vi "RPC Method Query.vi"(8 "error in (no error)":errorcluster, 11 "OOP Server in":refnum<class "Query Server.lvclass">) -> (0 "error out":errorcluster, 3 "OOP Server out":refnum<class "Query Server.lvclass">)   [LabVIEW 2016, in "Query Server.lvlib" / "Query Server.lvclass"]
uses:
  Query Server.lvclass
  RPC Messages/QueryResponse/QueryResponse_Data.ctl
panel:
  out "State Data":string
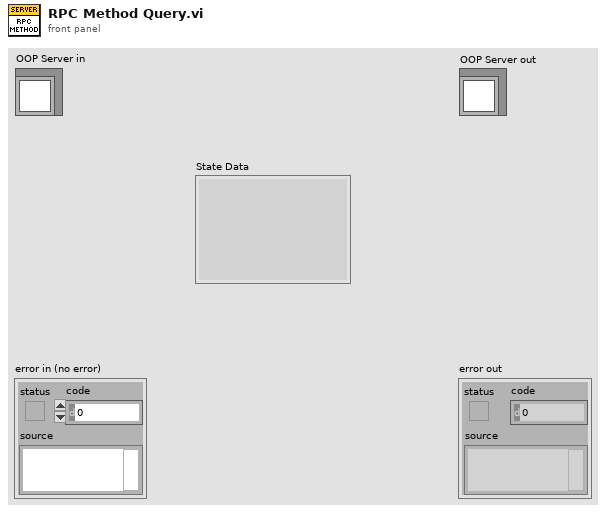
[diagram p1: front panel]
types:
  T1 = typedef "Query Server.lvlib/Query Server.lvclass/QueryResponse_Data.ctl" = cluster{"message":string, "status":i32}
  T2 = typedef "Query Server.lvlib/Query Server.lvclass/Server Internal UEs.ctl" = cluster{"Invoke Internal UE":refnum<user-event>, "Query Internal UE":refnum<user-event>, "Register Internal UE":refnum<user-event>}
  T3 = typedef "Query Server.lvlib/Query Server.lvclass/Server gRPC UEs.ctl" = cluster{"Invoke gRPC UE":refnum<user-event>, "Query gRPC UE":refnum<user-event>, "Register gRPC UE":refnum<user-event>}
  T4 = typedef "Query Server.lvlib/gprc-lvsupport.lvlib/grpcId.ctl" = u64
  T5 = typedef "Query Server.lvlib/Query Server.lvclass/QueryRequest_Data.ctl" = cluster{"query":string}
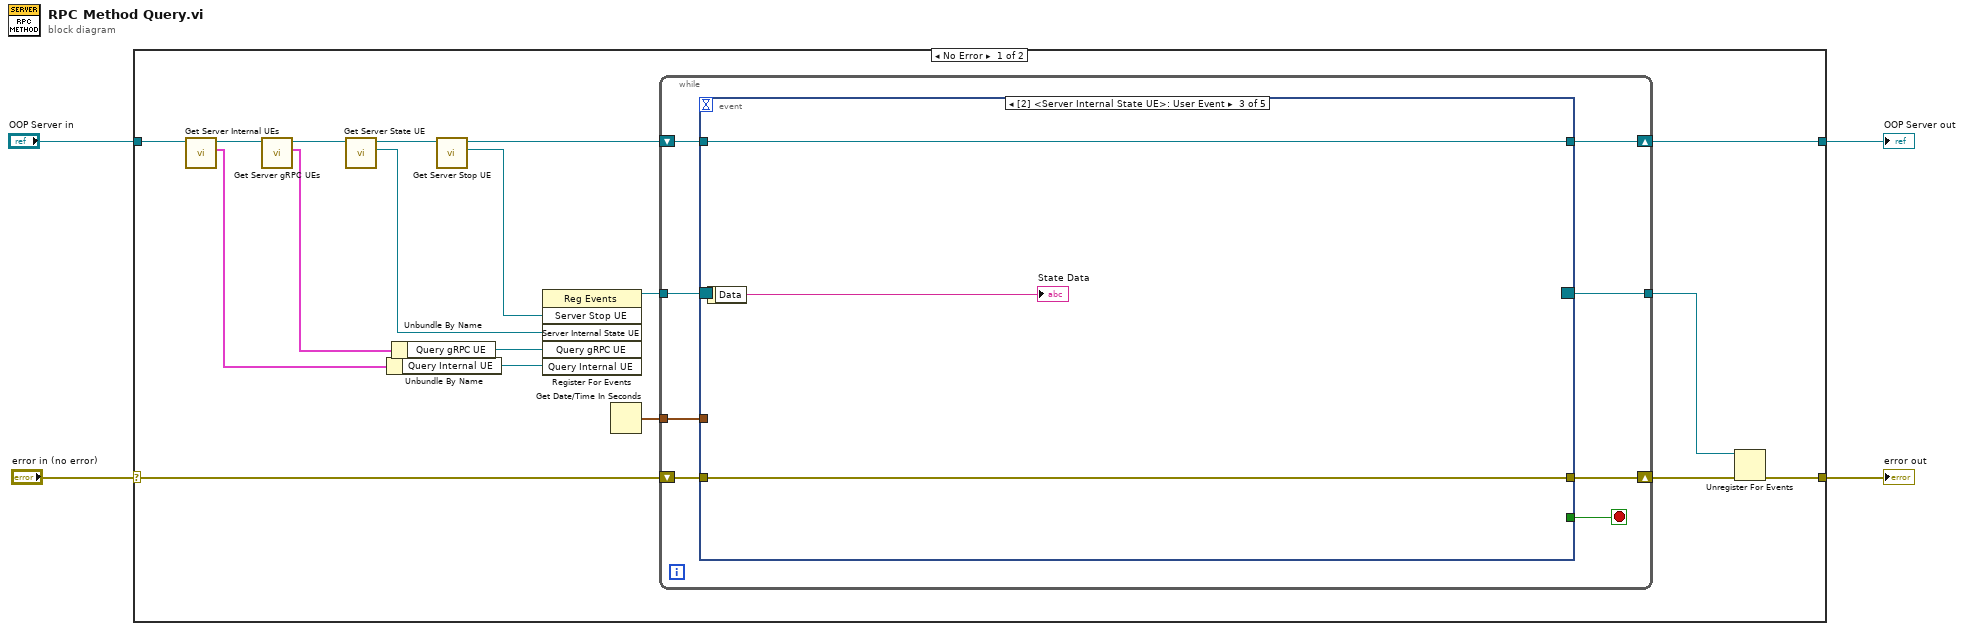
[diagram p0: block diagram]
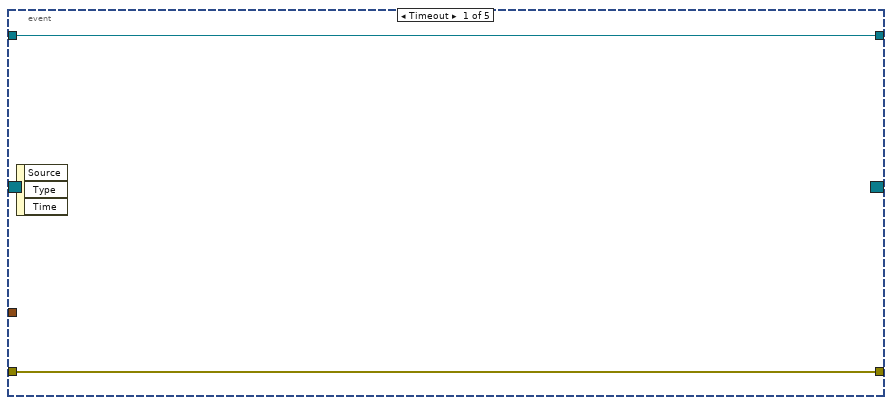
[diagram p2: hidden frame]
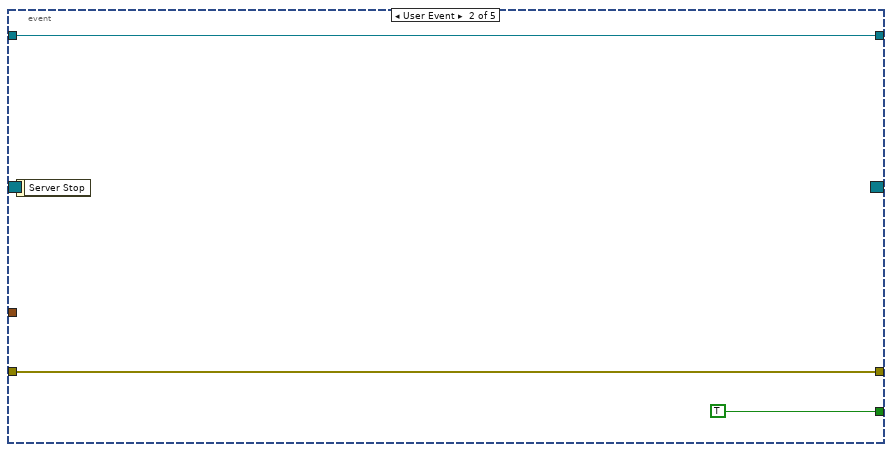
[diagram p3: hidden frame]
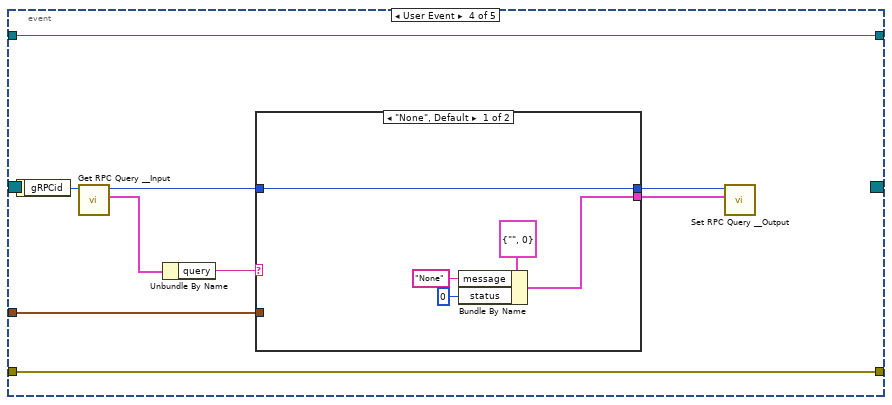
[diagram p4: hidden frame]
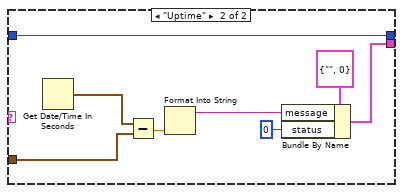
[diagram p5: hidden frame]
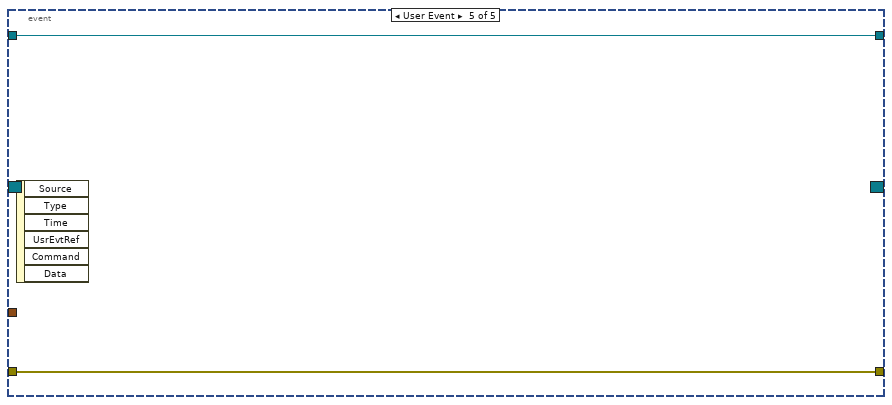
[diagram p6: hidden frame]
diagram:
  n1 = case shown="No Error" "error in (no error)" {
    selector: "error in (no error)" -> [w18 w64]
    tunnel: [w16 w64] -> w3
    tunnel: "OOP Server in" -> [w20 w63]
    tunnel: [w6 w63] -> w1
    frame No Error {
      n2 = call "Get Server Internal UEs.vi"("OOP Server in"=w20) -> ("Server Internal UEs"=w12:T2, "OOP Server out"=w19:refnum<class "Query Server.lvclass">)  [unwired: 9 in]
      n3 = call "Get Server gRPC UEs.vi"("OOP Server in"=w19) -> ("Server gRPC UEs"=w14:T3, "OOP Server out"=w9:refnum<class "Query Server.lvclass">)  [unwired: 8 in, 1 out]
      n4 = call "Get Server State UE.vi"("Template Server in"=w9) -> ("Server Internal State UE"=w7:refnum<user-event>, "Template Server out"=w8:refnum<class "Query Server.lvclass">)  [unwired: 9 in]
      n5 = Unbundle By Name ("Unbundle Internal UE")(w12) -> ("Query Internal UE"=w11:refnum<user-event>)
      n6 = Unbundle By Name ("Unbundle gRPC UE")(w14) -> ("Query gRPC UE"=w13:refnum<user-event>)
      n7 = call "Get Server Stop UE.vi"("OOP Server in"=w8) -> ("Server Stop UE"=w22:refnum<user-event>, "OOP Server out"=w10:refnum<class "Query Server.lvclass">)  [unwired: 9 in]
      n8 = register-events(w22, w7, w13, w11) -> (reference out=w21:refnum<event-registration>)  [unwired: 2 in, 1 out]
      n9 = Get Date/Time In Seconds() -> (seconds since 1Jan1904=w5:timestamp)
      n10 = while {
        tunnel: w21 -> [w30]
        tunnel: [w26] -> w15
        shift-right: [w27] -> w17
        shift-left: w18 -> [w28]
        shift-right: [w24] -> w6
        shift-left: w10 -> [w25]
        tunnel: w5 -> [w23]
        stop <- w29 stop-if-true
        n11 = event "RPC Method Event Structure" shown="[2] <Server Internal State UE>: User Event" {
          selector: w30 -> [_ _ _ _ _]
          dyn-events: [_ _ _ _ _] -> w26
          timeout: _ -> [_ _ _ _ _]
          tunnel: [_ TRUE _ _ _] -> w29
          tunnel: w28 -> [w32 w34 w38 w47 w62]
          tunnel: [w32 w34 w38 w47 w62] -> w27
          tunnel: w25 -> [w31 w33 w37 w46 w61]
          tunnel: [w31 w33 w37 w46 w61] -> w24
          tunnel: w23 -> [_ _ _ w39 _]
          event Timeout {
            n12 = event-data() -> ()  [unwired: 1 in, 3 out]
          }
          event User Event {
            n13 = event-data() -> ()  [unwired: 1 in, 1 out]
          }
          event User Event {
            n14 = event-data() -> ("Data"=→"State Data":string)  [unwired: 1 in]
          }
          event User Event {
            n15 = event-data() -> ("gRPCid"=w45:T4)  [unwired: 1 in]
            n16 = call "Get RPC Query __Input.vi"("gRPCid in"=w45) -> ("Message Data"=w44:T5, "gRPCid out"=w42:T4)  [unwired: 8 in, 1 out]
            n17 = Unbundle By Name(w44) -> ("query"=w43:string)
            n18 = case shown="\"None\", Default" w43 {
              tunnel: w42 -> [w52 w60]
              tunnel: [w52 w60] -> w41
              tunnel: [w48 w55] -> w40
              tunnel: w39 -> [_ w54]
              frame "None", Default {
                n19 = Bundle By Name(cluster=T1 {"message"="", "status"=0} ("Message Data"), "message"="None", "status"=0) -> (w48:T1)
              }
              frame "Uptime" {
                n20 = Get Date/Time In Seconds() -> (seconds since 1Jan1904=w59:timestamp)
                n21 = Subtract(x=w59, y=w54) -> (x-y=w58:dbl)
                n22 = Format Into String(w58) -> (resulting string=w53:string)  [unwired: 3 in, 1 out]
                n23 = Bundle By Name(cluster=T1 {"message"="", "status"=0} ("Message Data"), "message"=w53, "status"=0) -> (w55:T1)
              }
            }
            n24 = call "Set RPC Query __Output.vi"("Message Data"=w40, "gRPCid in"=w41) -> ()  [unwired: 9 in, 1 out]
          }
          event User Event {
            n25 = event-data() -> ()  [unwired: 1 in, 6 out]
          }
        }
      }
      n26 = Unregister For Events(event registration refnum=w15, error in=w17) -> (error out=w16:errorcluster)
    }
    frame Error {
    }
  }
  "error out" <- w3
  "OOP Server out" <- w1
